vi "AssetMgrCreateDeviceFromHardwareRequest_Parse.vi"(8 "error in (no error)":errorcluster, 11 "Message":T14) -> (0 "error out":errorcluster, 1 "Body":T1, 2 "Header":T13, 3 "AssetMgrCreateDeviceFromHardwareRequest":T12)   [LabVIEW 2017]
uses:
  <vilib>/addons/InsightCM/MessageBus/Base/controls/Message.ctl
  <vilib>/addons/InsightCM/MessageBus/Base/controls/MessageHeader.ctl
  <vilib>/addons/InsightCM/MessageBus/Base/controls/KeyValuePair.ctl
  <vilib>/addons/InsightCM/MessageBus/MessageLibrary/AssetManager/controls/AssetMgrCreateDeviceFromHardwareRequest.ctl
  <vilib>/addons/InsightCM/MessageBus/MessageLibrary/AssetManager/controls/AssetMgrCreateDeviceFromHardwareRequestBody.ctl
  <vilib>/addons/InsightCM/MessageBus/Base/controls/Device.ctl
  <vilib>/addons/InsightCM/MessageBus/Base/controls/DeviceState.ctl
  <vilib>/addons/InsightCM/MessageBus/Base/controls/DataGroup.ctl
  <vilib>/addons/InsightCM/MessageBus/Base/controls/BurstModeTrigger.ctl
  <vilib>/addons/InsightCM/MessageBus/Base/controls/Trigger.ctl
  <vilib>/addons/InsightCM/MessageBus/Base/controls/Condition.ctl
  <vilib>/addons/InsightCM/MessageBus/Base/controls/DeviceSensorGroup.ctl
  <vilib>/addons/InsightCM/MessageBus/Base/controls/WirelessEndpoint.ctl
  <vilib>/addons/InsightCM/MessageBus/Base/controls/WirelessChannel.ctl
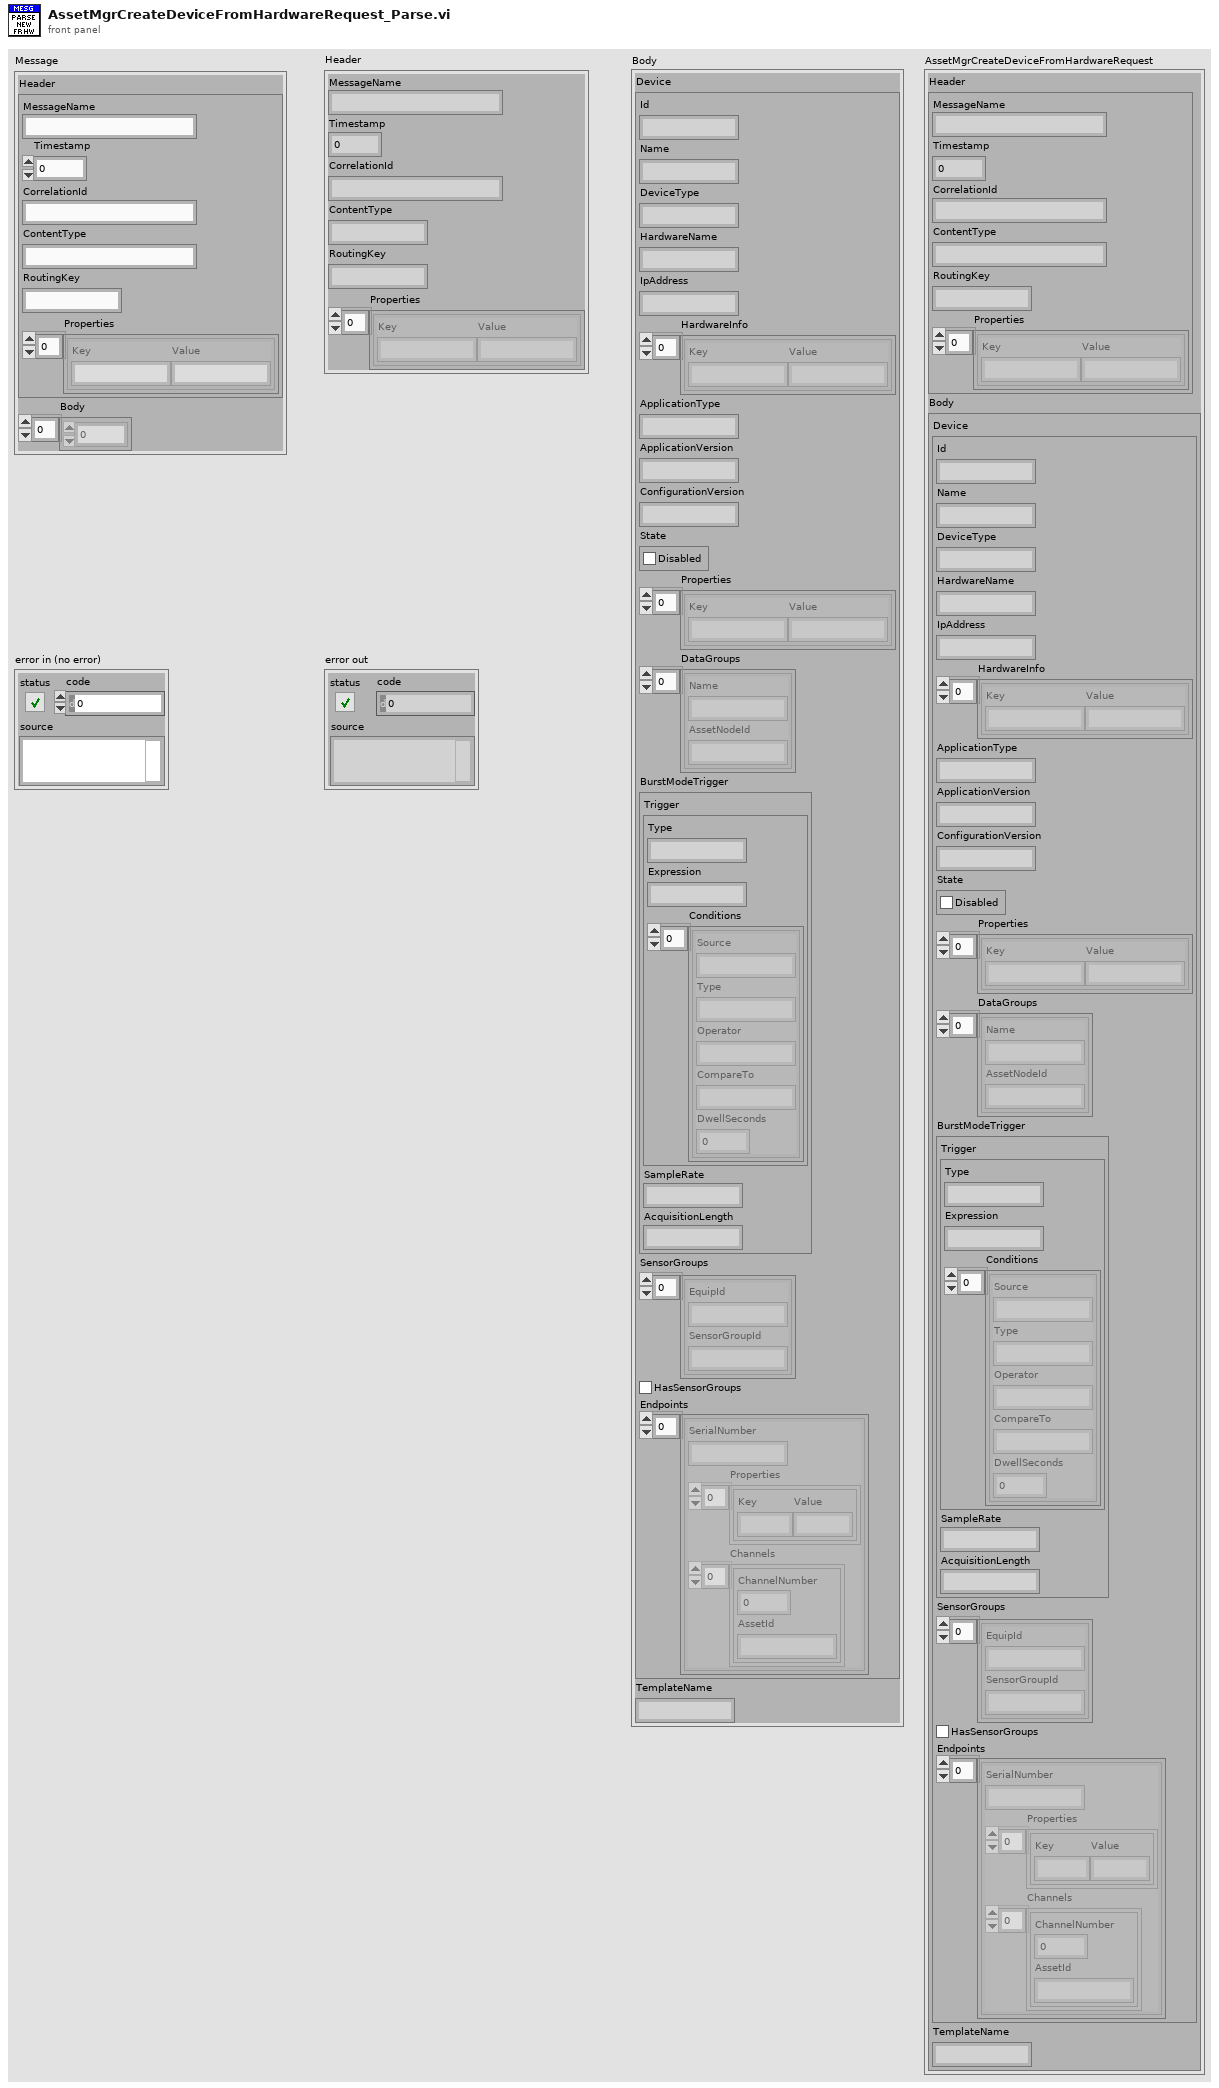
[diagram p1: front panel]
types:
  T1 = typedef "AssetMgrCreateDeviceFromHardwareRequestBody.ctl" = cluster{"Device":T2, "TemplateName":string}
  T2 = typedef "Device.ctl" = cluster{"Id":string, "Name":string, "DeviceType":string, "HardwareName":string, "IpAddress":string, "HardwareInfo":T3[], "ApplicationType":string, "ApplicationVersion":string, "ConfigurationVersion":string, "State":T4, "Properties":T3[], "DataGroups":T5[], "BurstModeTrigger":T6, "SensorGroups":T9[], "HasSensorGroups":bool, "Endpoints":T10[]}
  T3 = typedef "KeyValuePair.ctl" = cluster{"Key":string, "Value":string}
  T4 = typedef "DeviceState.ctl" = cluster{"Disabled":bool}
  T5 = typedef "DataGroup.ctl" = cluster{"Name":string, "AssetNodeId":string}
  T6 = typedef "BurstModeTrigger.ctl" = cluster{"Trigger":T7, "SampleRate":string, "AcquisitionLength":string}
  T7 = typedef "Trigger.ctl" = cluster{"Type":string, "Expression":string, "Conditions":T8[]}
  T8 = typedef "Condition.ctl" = cluster{"Source":string, "Type":string, "Operator":string, "CompareTo":string, "DwellSeconds":dbl}
  T9 = typedef "DeviceSensorGroup.ctl" = cluster{"EquipId":string, "SensorGroupId":string}
  T10 = typedef "WirelessEndpoint.ctl" = cluster{"SerialNumber":string, "Properties":T3[], "Channels":T11[]}
  T11 = typedef "WirelessChannel.ctl" = cluster{"ChannelNumber":i32, "AssetId":string}
  T12 = typedef "AssetMgrCreateDeviceFromHardwareRequest.ctl" = cluster{"Header":T13, "Body":T1}
  T13 = typedef "MessageHeader.ctl" = cluster{"MessageName":string, "Timestamp":i64, "CorrelationId":string, "ContentType":string, "RoutingKey":string, "Properties":T3[]}
  T14 = typedef "Message.ctl" = cluster{"Header":T13, "Body":u8[]}
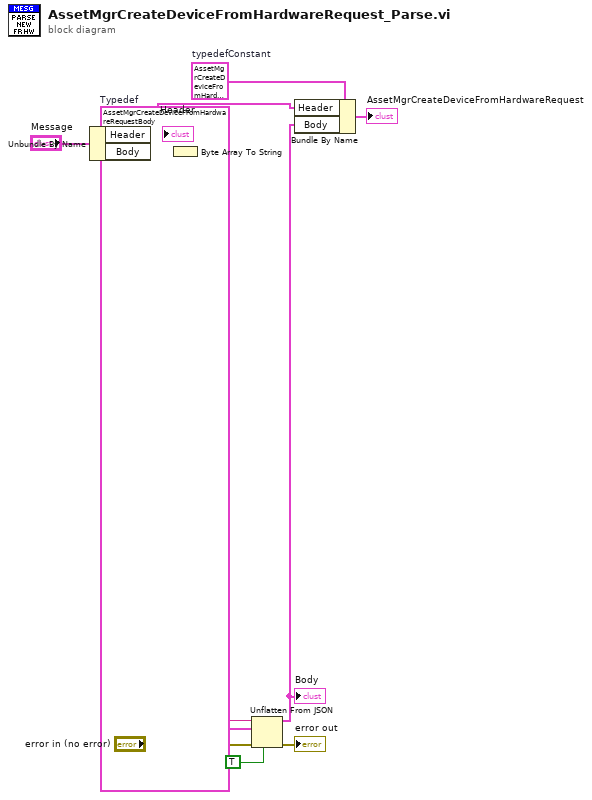
[diagram p0: block diagram]
diagram:
  w3 = T12 {"Header"={"MessageName"="", "Timestamp"=0, "CorrelationId"="", "ContentType"="", "RoutingKey"="", "Properties"=[]}, "Body"={"Device"={"Id"="", "Name"="", "DeviceType"="", "HardwareName"="", "IpAddress"="", "HardwareInfo"=[], "ApplicationType"="", "ApplicationVersion"="", "ConfigurationVersion"="", "State"={"Disabled"=FALSE}, "Properties"=[], "DataGroups"=[], "BurstModeTrigger"={"Trigger"={"Type"="", "Expression"="", "Conditions"=[]}, "SampleRate"="", "AcquisitionLength"=""}, "SensorGroups"=[], "HasSensorGroups"=FALSE, "Endpoints"=[]}, "TemplateName"=""}}  # typedefConstant
  w7 = T1 {"Device"={"Id"="", "Name"="", "DeviceType"="", "HardwareName"="", "IpAddress"="", "HardwareInfo"=[], "ApplicationType"="", "ApplicationVersion"="", "ConfigurationVersion"="", "State"={"Disabled"=FALSE}, "Properties"=[], "DataGroups"=[], "BurstModeTrigger"={"Trigger"={"Type"="", "Expression"="", "Conditions"=[]}, "SampleRate"="", "AcquisitionLength"=""}, "SensorGroups"=[], "HasSensorGroups"=FALSE, "Endpoints"=[]}, "TemplateName"=""}  # Typedef
  n1 = Unbundle By Name("Message") -> ("Header"=w9:T13, "Body"=w1:u8[])
  "Header" <- w9
  n2 = Byte Array To String(unsigned byte array=w1) -> (string=w6:string)
  n3 = Unflatten From JSON(JSON string=w6, type and defaults=w7, default null elements? (F)=TRUE, error in (no error)="error in (no error)") -> (value=w5:T1, error out=→"error out":errorcluster)  [unwired: 3 in]
  "Body" <- w5
  n4 = Bundle By Name(cluster=w3, "Header"=w9, "Body"=w5) -> (→"AssetMgrCreateDeviceFromHardwareRequest":T12)
